vi "Data_Recollection_GCFS.vi"(4 "error in (no error)":errorcluster, 6 "cnt":i32, 7 "Cluster":T2={"Core"={"Current VI Reference"=refnum, "Close Panel on Exit?"=FALSE}, "Your Boolean data"=FALSE, "Your string data"="", "Camera Cluster"={"Session"="", "Image"=refnum, "Position Image"=refnum, "PixelVal Image"=refnum, "Position Image Binary"=refnum, "Lable Image"=refnum, "Merged Image"=refnum}, "Data In Cluster"={"Images"={"Position Image path"=path "", "Sample folder path"=path "", "Rerun Folder path"=path "", "Rerun pos.img. path"=path ""}, "Sample Name"="", "Rerun Time"="", "Freezing value"=250.0, "Number of images"=0}, "Active"=FALSE, "Ready"=FALSE, "Exit"=FALSE, "Program_Start"="", "Data Out Cluster"={"Particle Measurements"=[], "Number of droplets"=0, "Time and temp"=[], "Sample time (YYYY-MM-DD_hh;mm)"=""}, "Load Rerun"=FALSE, "Rerun"=FALSE} {"Data Out Cluster"."Particle Measurements" format="%.2f"}) -> (0 "error out":errorcluster, 1 "Timestamp":string, 2 "Temp":dbl, 3 "Image Out":T1)   [LabVIEW 2024]
uses:
  RerunCluster_GCFS.ctl
  <vilib>/userDefined/High Color/IMAQdx.ctl
  <vilib>/vision/Image Controls.llb/IMAQ Image.ctl
panel:
  out "File Type out":string
  out "File Data Type out":i32
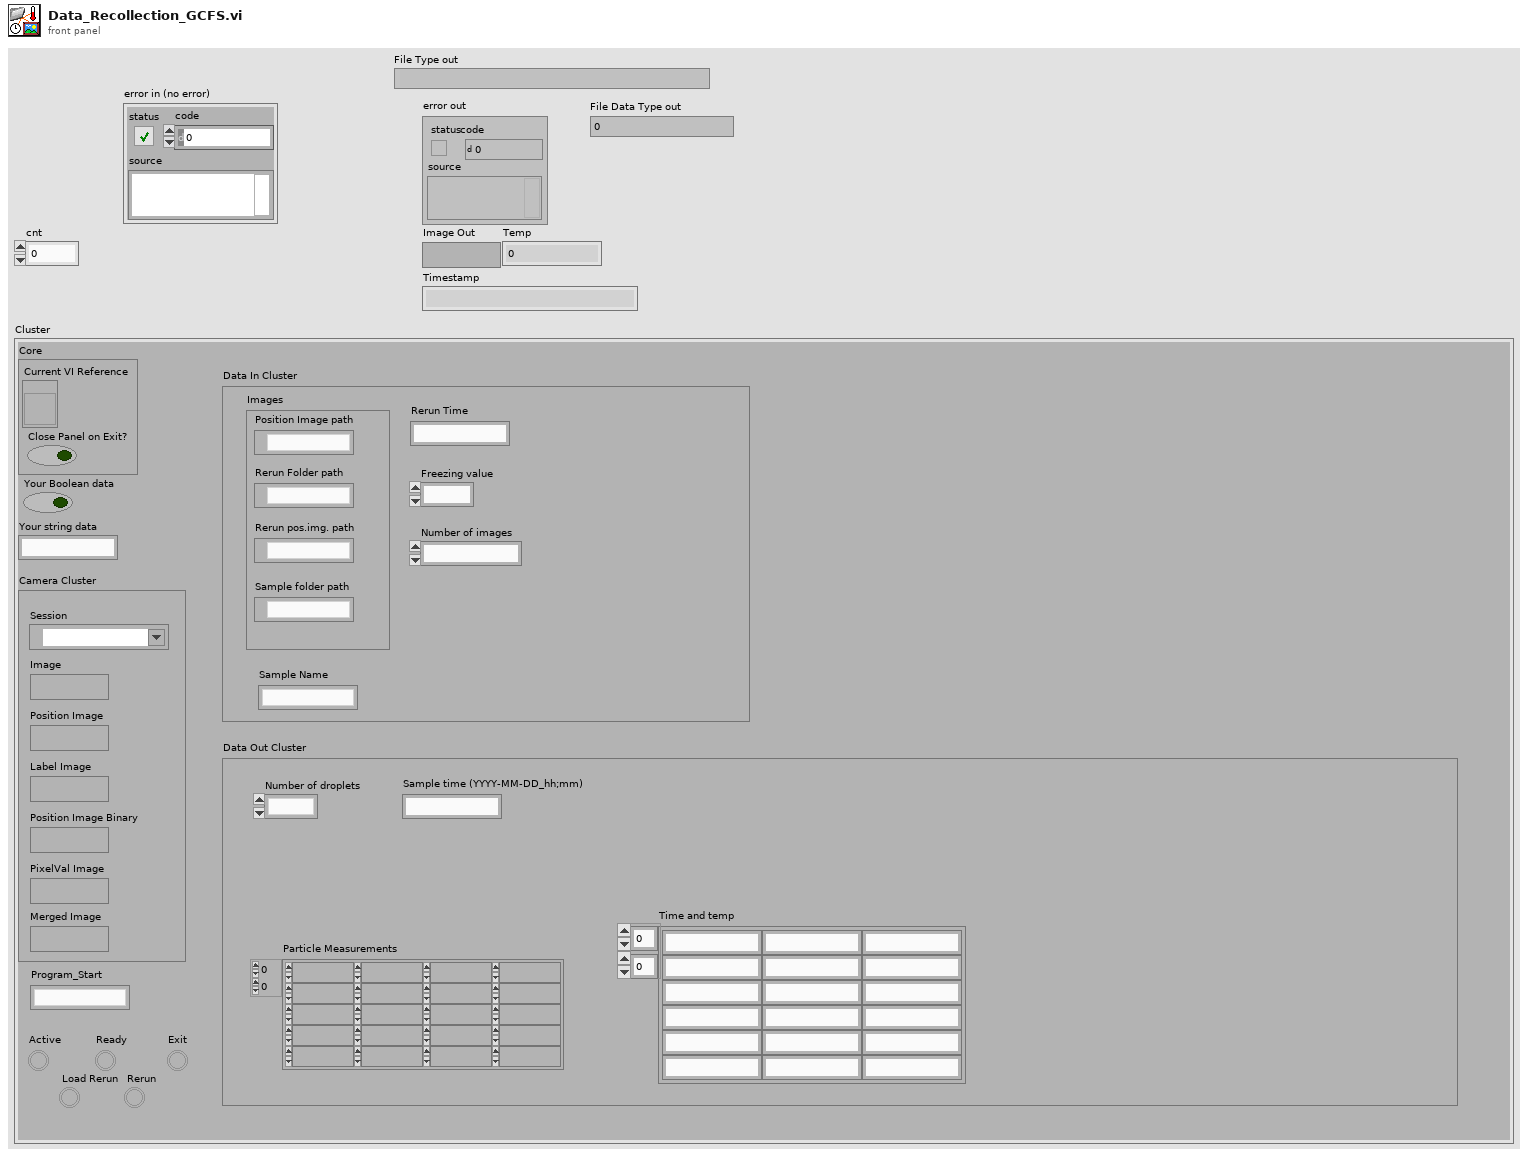
[diagram p1: front panel]
types:
  T1 = typedef "IMAQ Image.ctl" = refnum<image>
  T2 = typedef "RerunCluster_GCFS.ctl" = cluster{"Core":cluster{"Current VI Reference":refnum<vi>, "Close Panel on Exit?":bool}, "Your Boolean data":bool, "Your string data":string, "Camera Cluster":cluster{"Session":T3, "Image":T1, "Position Image":T1, "PixelVal Image":T1, "Position Image Binary":T1, "Lable Image":T1, "Merged Image":T1}, "Data In Cluster":cluster{"Images":cluster{"Position Image path":path, "Sample folder path":path, "Rerun Folder path":path, "Rerun pos.img. path":path}, "Sample Name":string, "Rerun Time":string, "Freezing value":sgl, "Number of images":i32}, "Active":bool, "Ready":bool, "Exit":bool, "Program_Start":string, "Data Out Cluster":cluster{"Particle Measurements":dbl[][], "Number of droplets":i32, "Time and temp":string[][], "Sample time (YYYY-MM-DD_hh;mm)":string}, "Load Rerun":bool, "Rerun":bool}
  T3 = typedef "IMAQdx.ctl" = refnum<k21>
  T4 = typedef "Image Type" = u32
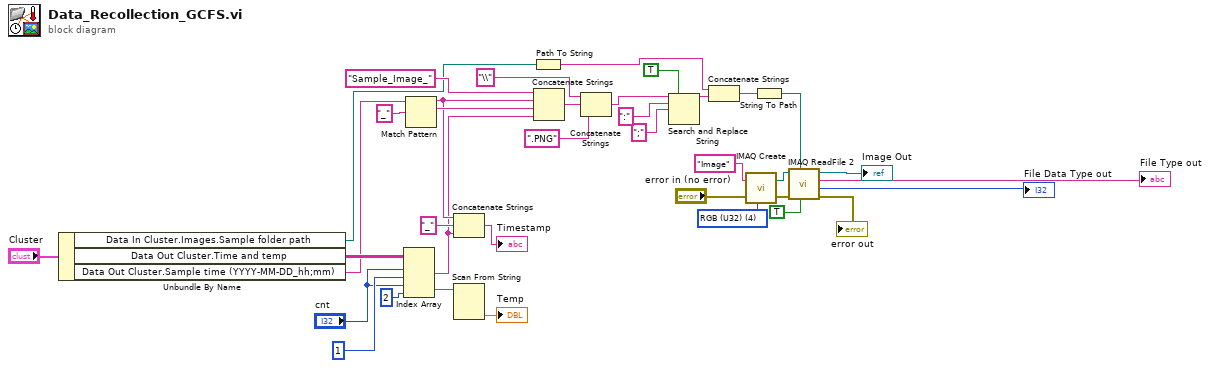
[diagram p0: block diagram]
diagram:
  w6 = T4 4 items=["Grayscale (U8)", "Grayscale (I16)", "Grayscale (SGL)", "Complex (CSG)", "RGB (U32)", "HSL (U32)", "RGB (U64)", "Grayscale (U16)"] ("Image Type")
  n1 = Unbundle By Name("Cluster") -> ("Data In Cluster.Images.Sample folder path"=w30:path, "Data Out Cluster.Time and temp"=w36:string[][], "Data Out Cluster.Sample time (YYYY-MM-DD_hh;mm)"=w34:string)
  n2 = Index Array(array=w36, index (row) #1="cnt", index (col) #1=1 ("disabled index (col)"), index (row) #2="cnt", index (col) #2=2 ("disabled index (col)")) -> (element #1=w25:string, element #2=w21:string)
  n3 = Match Pattern(string=w34, regular expression="_") -> (before substring=w27:string, match substring=w32:string)  [unwired: 1 in, 2 out]
  n4 = Concatenate Strings(w27, "_" ("string"), w25) -> (→"Timestamp":string)
  n5 = Scan From String(input string=w21) -> (output 1=→"Temp":dbl)  [unwired: 4 in, 3 out]
  n6 = Path To String(path=w30) -> (string=w11:string)
  n7 = Concatenate Strings("Sample_Image_" ("string"), w27, w32, w25) -> (w29:string)
  n8 = Concatenate Strings("\\" ("string"), w29, ".PNG" ("string")) -> (w17:string)
  n9 = Search and Replace String(replace all?=TRUE ("replace all? (F)"), input string=w17, search string=":", replace string=";" ("replace string (\"\")")) -> (result string=w13:string)  [unwired: 4 in, 3 out]
  n10 = Concatenate Strings(w11, w13) -> (w12:string)
  n11 = call "IMAQ Create"("Image Name"="Image", "Image Type"=w6, "error in (no error)"="error in (no error)") -> ("New Image"=w10:T1, "error out"=w7:errorcluster)  [unwired: 2 in]
  n12 = String To Path(string=w12) -> (path=w28:path)
  n13 = call "IMAQ ReadFile 2"("Use File Path Image Type"=TRUE, "File Path"=w28, "error in (no error)"=w7, "Image"=w10) -> ("error out"=→"error out":errorcluster, "File Data Type out"=→"File Data Type out":i32, "File Type out"=→"File Type out":string, "Image Out"=→"Image Out":T1)  [unwired: 3 in, 1 out]
